vi "Main.vi"() -> ()   [LabVIEW 2016]
uses:
  Typedef/INS Data.ctl
  <vilib>/FPGAPlugInAG/roboRIO/niLvFpga_Open_roboRIO.vi
  <vilib>/rvi/interface/common/dynamic/niFpgaDynamicAddResources.vi
  <vilib>/FPGAPlugInAG/Dynamic/niLvFpga_Reset_Dynamic.vi
  <vilib>/Utility/error.llb/Error Cluster From Error Code.vi
  <vilib>/rvi/errors/niLvFpgaAdjustHostInterfaceError.vi
  <vilib>/myRIO/Common/Instrument Driver Framework/Utilities/vis/FPGA Ref Manager.vi
  <vilib>/myRIO/Common/Instrument Driver Framework/Utilities/vis/Ref Counter.vi
  <vilib>/FPGAPlugInAG/Dynamic/niLvFpga_Run_Dynamic.vi
  Shared resoruces/gear.vi
  Shared resoruces/Front Panel Control Variables.vi
  <vilib>/rvi/interface/nirviOpenFPGA/nirviOpenFPGA.xnode
  FPGA Bitfiles/AutoBikeMainFPGAbitfile.lvbitx
  <vilib>/rvi/interface/nirviMethod/nirviMethod.xnode
  <vilib>/rvi/interface/nirviReadWriteControl/nirviReadWriteControl.xnode
  <vilib>/rvi/interface/Simulation/niFpgaSimulationCallBeginRW.vi
  NiFpgaLv.dll
  <vilib>/myRIO/Instrument Drivers/Utilities/Utilities.lvlib
  Shared resoruces/Shared resources RT.lvlib
panel:
  in  "resetPID":bool
  in  "Reset Errors":bool
  in  "Send vel":bool
  in  "VEL":u16=850
  in  "UseGPS":bool
  in  "Gear":enum16{"7", "6", "5", "4", "3", "2", "1"}(ring)=enum."4"
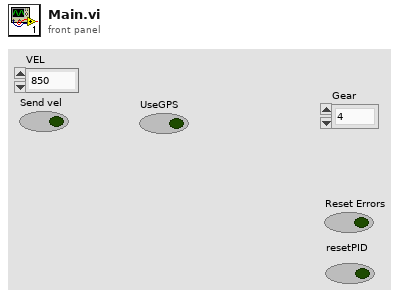
[diagram p1: front panel]
types:
  T1 = typedef "INS Data.ctl" = cluster{"Yaw":sgl, "Pitch":sgl, "Roll":sgl, "Lat":dbl, "Long":dbl, "Alt":dbl, "North":dbl, "East":dbl, "Down":dbl, "PosU":dbl, "VelU":dbl}
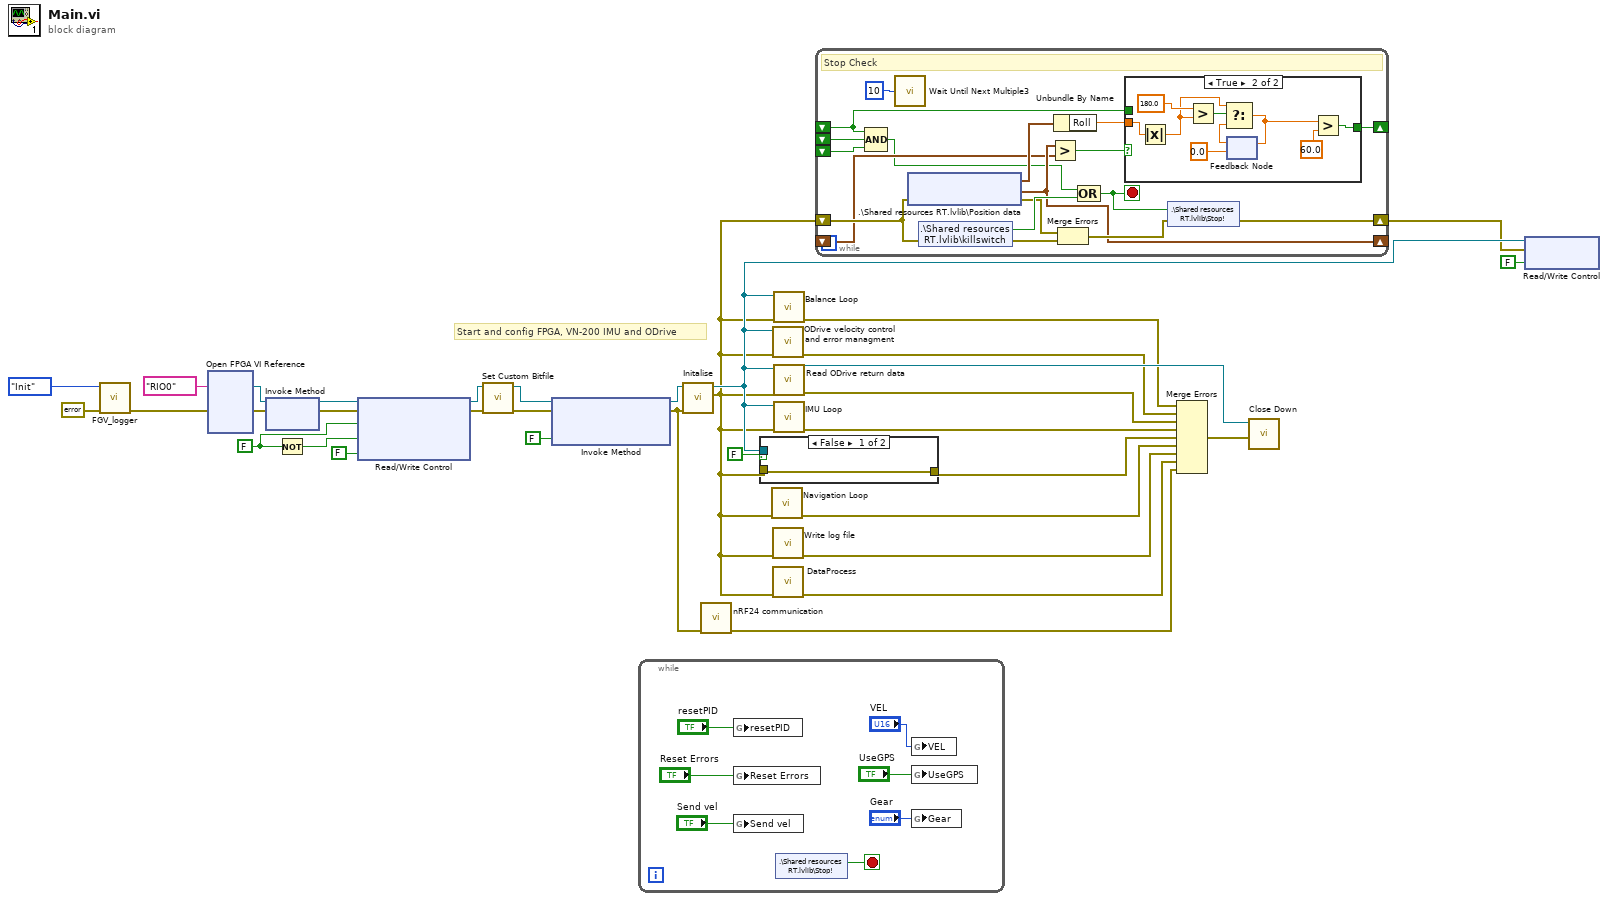
[diagram p0: block diagram]
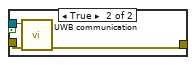
[diagram p2: hidden frame]
diagram:
  w25 = FALSE ("Steering motor on?")
  # "Start and config FPGA, VN-200 IMU and ODrive"
  n1 = call "FGV_logger.vi"("error in"=errorcluster {"status"=FALSE, "code"=0, "source"=""}, "Command"=enum16{"Update", "Log", "Init"}."Init") -> ("error out"=w31:errorcluster)  [unwired: 9 in]
  n2 = xnode "Open FPGA VI Reference"("error in"=w31, "resource name"=tag "RIO0") -> ("FPGA VI Reference Out"=w16:refnum<k20>, "error out"=w17:errorcluster)
  n3 = xnode "Invoke Method"("FPGA VI Reference In"=w16, "error in"=w17) -> ("FPGA VI Reference Out"=w29:refnum<k20>, "error out"=w28:errorcluster)
  n4 = Not(x=w25) -> (.not. x?=w26:bool)
  n5 = xnode "Read/Write Control"("FPGA VI Reference In"=w29, "error in"=w28, "Comm LED Green"=w25, "Comm LED Red"=w26, "MotorsON"=FALSE ("Rear wheel motor OFF?")) -> ("FPGA VI Reference Out"=w22:refnum<k20>, "error out"=w23:errorcluster)
  n6 = call <vilib>:"Set Custom Bitfile.vi"("error in (no error)"=w23, "Custom FPGA Reference In"=w22) -> ("error out"=w21:errorcluster, "Custom FPGA Reference Out"=w20:refnum<k20>)  [unwired: 8 in]
  n7 = xnode "Invoke Method"("FPGA VI Reference In"=w20, "error in"=w21, "Wait Until Done (F)"=FALSE) -> ("FPGA VI Reference Out"=w18:refnum<k20>, "error out"=w19:errorcluster)
  n8 = while {
    stop <- w35 stop-if-true
    n9 = global write "Front Panel Control Variables.vi" "resetPID"("resetPID") -> ()
    n10 = global write "Front Panel Control Variables.vi" "Reset Errors"("Reset Errors") -> ()
    n11 = global write "Front Panel Control Variables.vi" "Send vel"("Send vel") -> ()
    n12 = shared-variable ".\\Shared resources RT.lvlib\\Stop!"() -> (w35:bool)  [unwired: 1 in, 1 out]
    n13 = global write "Front Panel Control Variables.vi" "VEL"("VEL") -> ()
    n14 = global write "Front Panel Control Variables.vi" "UseGPS"("UseGPS") -> ()
    n15 = global write "gear.vi" "Gear"("Gear") -> ()
  }
  n16 = call "Initalise.vi"("error in (no error)"=w19, "FPGA Interface"=w18) -> ("Error out"=w4:errorcluster, "FPGA VI Reference Out"=w6:refnum<k20>)  [unwired: 7 in, 1 out]
  n17 = call "nRF24 communication.vi"("error in (no error)"=w19) -> ("error out"=w3:errorcluster)  [unwired: 10 in]
  n18 = case shown="False" FALSE {
    tunnel: [w42 w45] -> w10
    tunnel: w6 -> [_ w44]
    tunnel: w4 -> [w42 w43]
    frame False {
    }
    frame True {
      n19 = call "UWB communication.vi"("error in (no error)"=w43, "FPGA VI Reference In"=w44) -> ("error out"=w45:errorcluster)  [unwired: 8 in, 1 out]
    }
  }
  n20 = call "Navigation Loop.vi"("error in (no error)"=w4) -> ("error out"=w9:errorcluster)  [unwired: 10 in]
  n21 = call "ODrive velocity control and error managment.vi"("error in (no error)"=w4, "Refnum in"=w6) -> ("Error out"=w13:errorcluster)  [unwired: 8 in, 1 out]
  n22 = call "Write log file.vi"("error in (no error)"=w4) -> ("error out"=w8:errorcluster)  [unwired: 10 in]
  n23 = call "DataProcess.vi"("error in (no error)"=w4) -> ("error out"=w2:errorcluster)  [unwired: 10 in]
  n24 = call "Balance Loop.vi"("error in (no error)"=w4, "Refnum in"=w6) -> ("error out"=w14:errorcluster)  [unwired: 8 in, 1 out]
  n25 = call "Read ODrive return data.vi"("error in (no error)"=w4, "Refnum in"=w6) -> ("error out"=w12:errorcluster, "Refnum out"=w15:refnum<k20>)  [unwired: 8 in]
  n26 = call "IMU Loop.vi"("error in (no error)"=w4, "FPGA ref in"=w6) -> ("error out"=w11:errorcluster)  [unwired: 9 in]
  n27 = while {
    shift-right: [w63] -> w5
    shift-left: w4 -> [w59]
    shift-right: [w54] -> _
    shift-left: _ -> [w53]
    shift-right: [w50] -> _
    shift-left: _ -> [w48]
    shift-left: _ -> [w49]
    shift-left: _ -> [w47]
    stop <- w56 stop-if-true
    # "Stop Check"
    n28 = Compound Arithmetic op=AND(w48, w49, w47) -> (w46:bool)
    n29 = call "Wait Until Next Multiple3"("Count(mSec)"=u32 10) -> ()  [unwired: 1 out]
    n30 = shared-variable ".\\Shared resources RT.lvlib\\Position data"(error in=w59) -> (w57:T1, error out=w58:errorcluster, w54:timestamp)
    n31 = shared-variable ".\\Shared resources RT.lvlib\\killswitch"(error in=w59) -> (w62:bool, error out=w60:errorcluster)
    n32 = Greater?(x=w54, y=w53) -> (0:w52:bool)
    n33 = Unbundle By Name(w57) -> ("Roll"=w51:sgl)
    n34 = Merge Errors(w58, w60) -> (w61:errorcluster)
    n35 = Compound Arithmetic op=OR(w46, w62) -> (w56:bool)
    n36 = case shown="True" w52 {
      tunnel: w51 -> [_ w67]
      tunnel: [w64 w72] -> w50
      tunnel: w48 -> [w64 _]
      frame False {
      }
      frame True {
        n37 = Absolute Value(x=w67) -> (abs(x)=w66:sgl)
        n38 = Greater?(x=sgl 180.0 ("upper limit"), y=w66) -> (0:w71:bool)
        n39 = feedback #1(sgl 0.0 ("Roll")) -> (w69:sgl)
        n40 = Select(t=w66, s=w71, f=w69) -> (s? t:f=w65:sgl)
        n41 = feedback-in #1(w65) -> ()
        n42 = Greater?(x=w65, y=sgl 60.0) -> (0:w72:bool)
      }
    }
    n43 = shared-variable ".\\Shared resources RT.lvlib\\Stop!"(w56, error in=w61) -> (error out=w63:errorcluster)
  }
  n44 = Merge Errors(w14, w13, w12, w11, w10, w9, w8, w2, w3) -> (w33:errorcluster)
  n45 = call "Close Down.vi"("error in (no error)"=w33, "FPGA Interface"=w15) -> ()  [unwired: 9 in, 1 out]
  n46 = xnode "Read/Write Control"("FPGA VI Reference In"=w6, "error in"=w5, "MotorsON"=FALSE) -> ()  [unwired: 2 out]
